vi "MCL Single Write Z.vi"(10 "handle":i32, 11 "position":dbl) -> (3 "function return":i32)   [LabVIEW 2017, in "Madlib.lvlib"]
doc: "MADLIB_API int MCL_SingleWriteZ(double position, int handle);"
uses:
  Madlib.lvlib
  Madlib.dll
panel:
  out "error out":errorcluster
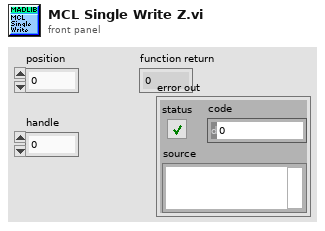
[diagram p1: front panel]
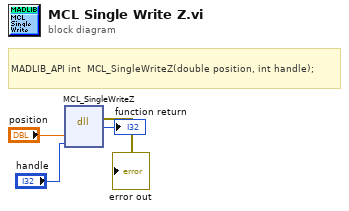
[diagram p0: block diagram]
diagram:
  # "MADLIB_API\tint\t\tMCL_SingleWriteZ(double position, int handle);"
  n1 = dll-call lib="C:/Users/Fred/dev/pump-probe/Piezo/lvlib/Madlib.*" fn="MCL_SingleWriteZ"("position"="position", "handle"="handle") -> (error out=→"error out":errorcluster, →"function return":i32)  [unwired: 5 in, 1 out]
